vi "ReinitializeWhenStopped.vi"(11 "JoystickValue":dbl) -> (3 "reinitialize? (F)":bool)   [LabVIEW 2013]
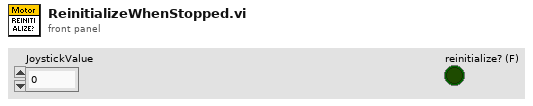
[diagram p1: front panel]
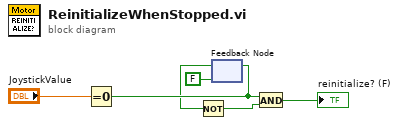
[diagram p0: block diagram]
diagram:
  n1 = Equal To 0?(x="JoystickValue") -> (x = 0?=w6:bool)
  n2 = feedback #1(FALSE ("Boolean")) -> (w1:bool)
  n3 = Not(x=w1) -> (.not. x?=w3:bool)
  n4 = feedback-in #1(w6) -> ()
  n5 = And(x=w6, y=w3) -> (x .and. y?=→"reinitialize? (F)":bool)
